vi "append_results_bundle.vi"(8 "Y":T1, 10 "X":T1) -> (2 "concat(X,Y)":T1)   [LabVIEW 2017]
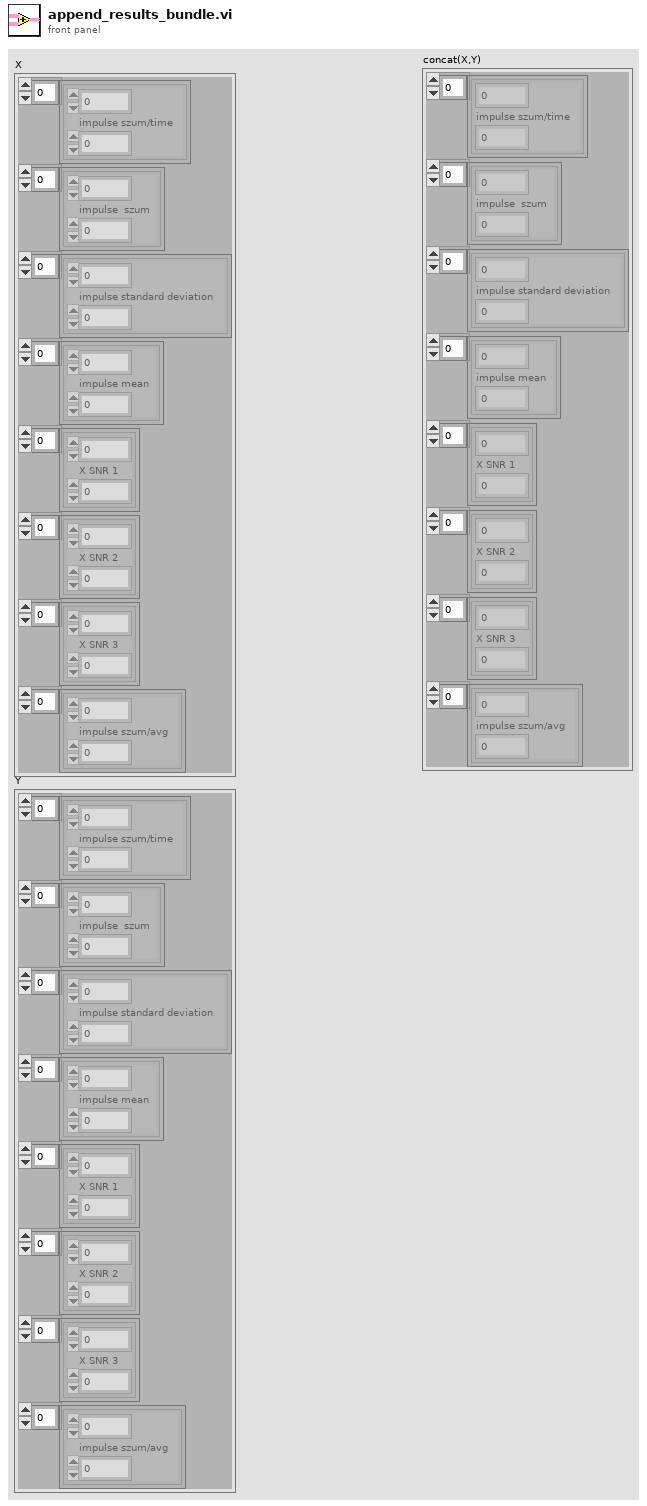
[diagram p1: front panel]
types:
  T1 = cluster{cluster{dbl, "impulse szum/time":dbl}[], cluster{dbl, "impulse  szum":dbl}[], cluster{dbl, "impulse standard deviation":dbl}[], cluster{dbl, "impulse mean":dbl}[], cluster{dbl, "X SNR 1":dbl}[], cluster{dbl, "X SNR 2":dbl}[], cluster{dbl, "X SNR 3":dbl}[], cluster{dbl, "impulse szum/avg":dbl}[]}
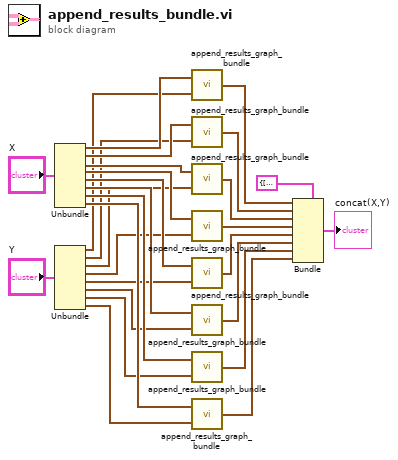
[diagram p0: block diagram]
diagram:
  n1 = Unbundle("X") -> (w16:cluster{dbl, "impulse szum/time":dbl}[], w15:cluster{dbl, "impulse  szum":dbl}[], w14:cluster{dbl, "impulse standard deviation":dbl}[], w13:cluster{dbl, "impulse mean":dbl}[], w12:cluster{dbl, "X SNR 1":dbl}[], w11:cluster{dbl, "X SNR 2":dbl}[], w10:cluster{dbl, "X SNR 3":dbl}[], w9:cluster{dbl, "impulse szum/avg":dbl}[])
  n2 = Unbundle("Y") -> (w8:cluster{dbl, "impulse szum/time":dbl}[], w7:cluster{dbl, "impulse  szum":dbl}[], w6:cluster{dbl, "impulse standard deviation":dbl}[], w5:cluster{dbl, "impulse mean":dbl}[], w4:cluster{dbl, "X SNR 1":dbl}[], w3:cluster{dbl, "X SNR 2":dbl}[], w2:cluster{dbl, "X SNR 3":dbl}[], w1:cluster{dbl, "impulse szum/avg":dbl}[])
  n3 = call "append_results_graph_bundle.vi"("Y"=w8, "X"=w16) -> ("concat(X,Y)"=w22:cluster{dbl, dbl}[])
  n4 = call "append_results_graph_bundle.vi"("Y"=w7, "X"=w15) -> ("concat(X,Y)"=w28:cluster{dbl, dbl}[])
  n5 = call "append_results_graph_bundle.vi"("Y"=w6, "X"=w14) -> ("concat(X,Y)"=w27:cluster{dbl, dbl}[])
  n6 = call "append_results_graph_bundle.vi"("Y"=w5, "X"=w13) -> ("concat(X,Y)"=w26:cluster{dbl, dbl}[])
  n7 = call "append_results_graph_bundle.vi"("Y"=w4, "X"=w12) -> ("concat(X,Y)"=w25:cluster{dbl, dbl}[])
  n8 = call "append_results_graph_bundle.vi"("Y"=w3, "X"=w11) -> ("concat(X,Y)"=w24:cluster{dbl, dbl}[])
  n9 = call "append_results_graph_bundle.vi"("Y"=w2, "X"=w10) -> ("concat(X,Y)"=w23:cluster{dbl, dbl}[])
  n10 = call "append_results_graph_bundle.vi"("Y"=w1, "X"=w9) -> ("concat(X,Y)"=w21:cluster{dbl, dbl}[])
  n11 = Bundle(cluster=T1 {[], [], [], [], [], [], [], []}, w22, w28, w27, w26, w25, w24, w23, w21) -> (→"concat(X,Y)":T1)
